vi "Destroy.vi"(8 "error in":errorcluster, 11 "UI_Manager in":refnum<class "UI_Library.lvclass">) -> (0 "error out":errorcluster, 3 "UI_Manager out":refnum<class "UI_Library.lvclass">)   [LabVIEW 2018, in "UI_Library.lvlib" / "UI_Library.lvclass"]
doc: "Destroy queue reference and cleanup all Controls references"
uses:
  UI_Library.lvclass
  UI_Library.lvclass/UI_Library.ctl
  <vilib>/Utility/Data Type/Type Definitions/Data Type.ctl
  <vilib>/Utility/Data Type/NI_Data Type.lvlib
  Controls/UI_RefCluster.ctl
  UI_Library.lvlib
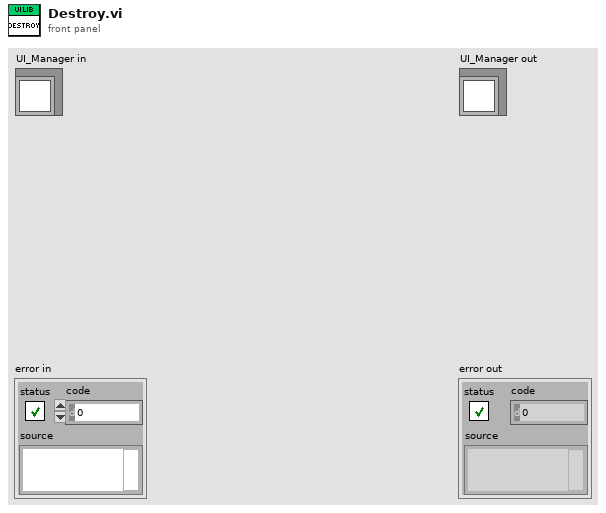
[diagram p1: front panel]
types:
  T1 = typedef "UI_Library.lvlib/UI_RefCluster.ctl" = cluster{"UI Ctrl Names":string[], "UI Ctrl DataType":T2[], "UI Ctrl Refs":refnum<vi>[]}
  T2 = typedef "NI_Data Type.lvlib/Data Type.ctl" = enum8{"Invalid Type", "Void", "I8", "I16", "I32", "I64", "U8", "U16", "U32", "U64", "Single Float", "Double Float", "Extended Float", "Single Complex", "Double Complex", "Extended Complex", "Enum U8", "Enum U16", "Enum U32", "Enum U64", "Single Float With Unit", "Double Float With Unit", "Extended Float With Unit", "Single Complex with Unit", "Double Complex with Unit", "Extended Complex with Unit", "Boolean", "String", "Path", "Picture", "Tag", "Array", "Cluster", "Variant", "LV Variant", "Waveform", "Timestamp", "Digital Waveform", "Digital Data", "ExpressData", "Refnum", "External Data", "VI", "Poly VI", "LabVIEW Class Instance", "Fixed Point", "Set Collection", "Map Collection"}
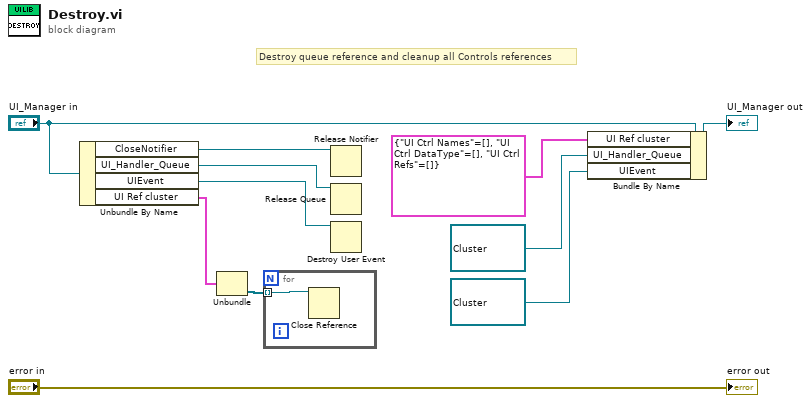
[diagram p0: block diagram]
diagram:
  # "Destroy queue reference and cleanup all Controls references"
  n1 = Unbundle By Name("UI_Manager in") -> ("CloseNotifier"=w1:refnum<notifier>, "UI_Handler_Queue"=w5:refnum<queue>, "UIEvent"=w4:refnum<user-event>, "UI Ref cluster"=w3:T1)
  n2 = Unbundle(w3) -> ("UI Ctrl Refs"=w2:refnum<vi>[])  [unwired: 2 out]
  n3 = for {
    tunnel: w2 -> [w12] mode=indexing
    n4 = Close Reference(reference=w12) -> ()  [unwired: 1 in, 1 out]
  }
  n5 = Release Notifier(notifier=w1) -> ()  [unwired: 2 in, 3 out]
  n6 = Release Queue(queue=w5) -> ()  [unwired: 2 in, 3 out]
  n7 = Destroy User Event(user event=w4) -> ()  [unwired: 1 in, 1 out]
  n8 = Bundle By Name(cluster="UI_Manager in", "UI Ref cluster"=T1 {"UI Ctrl Names"=[], "UI Ctrl DataType"=[], "UI Ctrl Refs"=[]}, "UI_Handler_Queue"=refnum<queue> refnum, "UIEvent"=refnum<user-event> refnum) -> (→"UI_Manager out":refnum<class "UI_Library.lvclass">)
  "error out" <- "error in"
